vi "Write Type.vi"(8 "error in (no error)":errorcluster, 10 "Type":enum16{"Secure", "Remove"}(ring), 11 "Secure Syringe in":refnum<class "SecureRelease Syringe.lvclass">) -> (0 "error out":errorcluster, 3 "Secure Syringe out":refnum<class "SecureRelease Syringe.lvclass">)   [LabVIEW 2020, in "SecureRelease Syringe.lvclass"]
uses:
  SecureRelease Syringe.lvclass
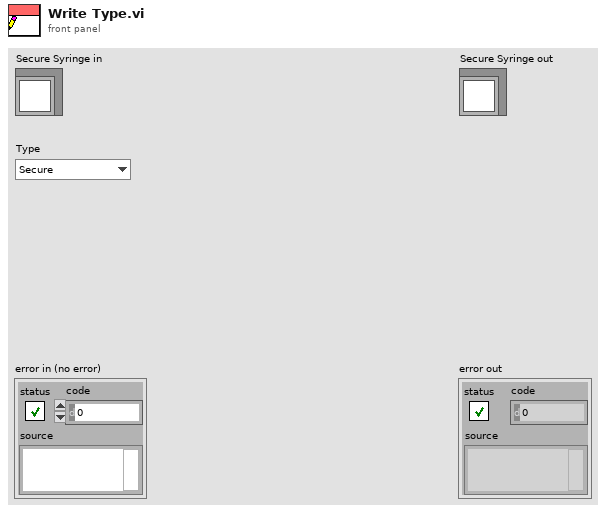
[diagram p1: front panel]
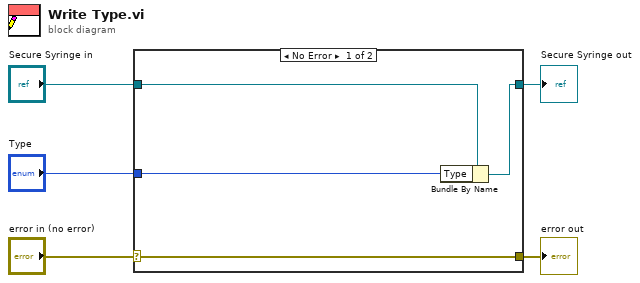
[diagram p0: block diagram]
diagram:
  n1 = case shown="No Error" "error in (no error)" {
    selector: "error in (no error)" -> [w9 w10]
    tunnel: [w9 w10] -> w4
    tunnel: [w7 w11] -> w2
    tunnel: "Secure Syringe in" -> [w8 w11]
    tunnel: "Type" -> [w6 _]
    frame No Error {
      n2 = Bundle By Name(cluster=w8, "Type"=w6) -> (w7:refnum<class "SecureRelease Syringe.lvclass">)
    }
    frame Error {
    }
  }
  "error out" <- w4
  "Secure Syringe out" <- w2
